vi "_LO_freq_Sweep_with_PM.vi"(9 "_LO_sweep":T3={"スケール"=200.0, "start (GHz)"=780.0, "stop (GHz)"=900.0, "step (GHz) "=0.1, "Wait(ms)"=10.0, "file_name"="", "パス"=path "", "measure"=0} {"measure" items=["SIS Current", "DMM34401A"]}, 10 "LO_misc":T1={"LO FRQ(GHz)"=900.0, "LO multi "=9.0, "LocK?"=FALSE, "LO REF multi"=4.0, "wait (ms)"=10.0, "SG Pow Min (dBm)"=10.0, "SG Pow Max (dBm)"=20.0, "SG Pow Step (dBm)"=0.2, "SGPow OPT? "=TRUE, "SG set frq"=25.0075, "SG set pow"=10.0}, 11 "Bias_LO_equip":T2={"Node address"=19, "CAN Interface"="CAN0", "Cartridge band"=10, "Slave Node in"={"Address"=19, "Serial Number"=[16, 71, 55, 76, 2, 8, 0, -15]}, "ObjHandle out"=159055936, "POL"=1, "sb"=1, "GPIB_SM (SIS S,V)"="24", "GPIB_DMM (SIS I)"="22", "GPIB_SM (MAG I) "="25", "GPIB_SG(LO)"="19", "GPIB_PW (PAMP) "="6", "GPIB_TMP1(8ch)"="12", "GPIB_TMP2(2ch)  "="13", "WCA_avg"=10, "Rsen"=10.0, "BiasModule"=0, "LOModule "=4, "WCA_LO_FREQ_SET"={"YTO Low freq. [GHz]"=14.42, "YTO High freq. [GHz]"=17.7, "Kvco"=1, "Lock Pol."=0, "SET LO FREQ"=72.5, "Multiplier"=6.0, "YTO (HEX)"=0, "YTO coarse( FREQ)"=25.0, "NULL PLL INTEGRATOR"=FALSE}} {"WCA_LO_FREQ_SET"."YTO coarse( FREQ)" min=25 max=150 step=0.0001 format="%.3f"; "WCA_LO_FREQ_SET"."Multiplier" min=3 max=6 step=3; "WCA_LO_FREQ_SET"."SET LO FREQ" min=25 max=150 step=0.0001 format="%.3f"; "WCA_LO_FREQ_SET"."Lock Pol." items=["Lower", "Upper"]; "WCA_LO_FREQ_SET"."Kvco" items=["7.5MHz/V", "15MHz/V"]; "WCA_LO_FREQ_SET"."YTO High freq. [GHz]" format="%.3f"; "WCA_LO_FREQ_SET"."YTO Low freq. [GHz]" format="%.3f"; "LOModule" items=["Manual Gunn+PAMP"=0, "B10Lab LO"=1, "WCA LO"=2, ""=3, "YIG発信器"=4, "none"=99]; "BiasModule" items=["B10Lab Bias"=0, "WCA BiasModule"=1, "none"=99]; "Slave Node in"."Serial Number" format="%.0x"; "Slave Node in"."Address" format="%.0x"; "Cartridge band" max=10 step=1; "Node address" format="%.0x"}) -> ()   [LabVIEW 2011]
uses:
  __sub_vi/WCA_NAOJ_sub_vi/WCA_Global.vi
panel:
  out "XYグラフ":cluster{dbl[], dbl[]}[](graph)
  in  "タブ制御器":enum32{"機器セッティング", "機器セッティング 2", "WCALOモニタ "}(tab)
  out "Link済み":bool
  out "error out":errorcluster={"status"=TRUE, "code"=-1074388991, "source"="NI-CAN Wait For State\n(ncWait.vi)"} caption="エラー出力"
  out "LO周波数":dbl=900.0
  out "出力":dbl=0.0096099853515625
  out "GET_PLL":T4={"PLL_ASSY_T"=37.887573, "PLL_REF_TOT_P"=-0.004119873, "PLL_IF_TOT_P"=0.010223389, "PLL_CORR_V"=0.08273038, "PLL_LOCK_V"=0.06496083, "PLL_5V_SUPPLY_V"=19.049072, "Temp_TF"=TRUE, "PLL Ref Pwr_TF"=FALSE, "IF Pwr_TF"=FALSE, "PLL Corr_TF"=TRUE, "PLL Lock V_TF"=FALSE, "PLL Nominal_TF"=FALSE}
  out "GET_AMC":T5={"AMC_A_DRAIN_V"=3.48938, "AMC_A_DRAIN_C"=64.42261, "AMC_A_GATE_V"=-0.4689026, "AMC_B_DRAIN_V"=4.34021, "AMC_B_DRAIN_C"=301.4679, "AMC_B_GATE_V"=-0.48934937, "AMC_E_DRAIN_V"=3.977356, "AMC_E_DRAIN_C"=342.6819, "AMC_E_GATE_V"=-0.24169922, "AMC_3V_SUPPLY_V"=-13.227844, "AMC_5V_MON"=5.204468, "AMC_MULT_D_V"=0.0}
  out "GET_PHOTOMIXER":T6={"PHOTMIX_ State"=enum."Disabled", "PHOTOMIX_BIAS_V"=-0.0012207031, "PHOTOMIX_BIAS_C"=-0.0032043457}
  out "GET_PA":T7={"PA_A_DRAIN_V"=4.0403748, "PA_A_DRAIN_C"=429.99268, "PA_A_GATE_V"=-0.00061035156, "PA_B_DRAIN_V"=0.0048828125, "PA_B_DRAIN_C"=2.5482178, "PA_B_GATE_V"=0.0015258789, "PA_3V_SUPPLY_V"=3.7130737, "PA_5V_MON"=5.3082275}
  # "LO freq. [GHz]"
  # "YTO LOW\n/High Freq."
  # "ZERO Intgrtr"
  # "Node Address"
  # "Serial Number"
  # "Vd [V]"
  # "Id [mA]"
  # "Vg [V]"
  # "AMC A"
  # "AMC B"
  # "AMC E"
  # "Vd [V]"
  # "Id [mA]"
  # "Vg [V]"
  # "PA -3V Supply"
  # "-3V"
  # "PA A"
  # "+5V"
  # "PA B"
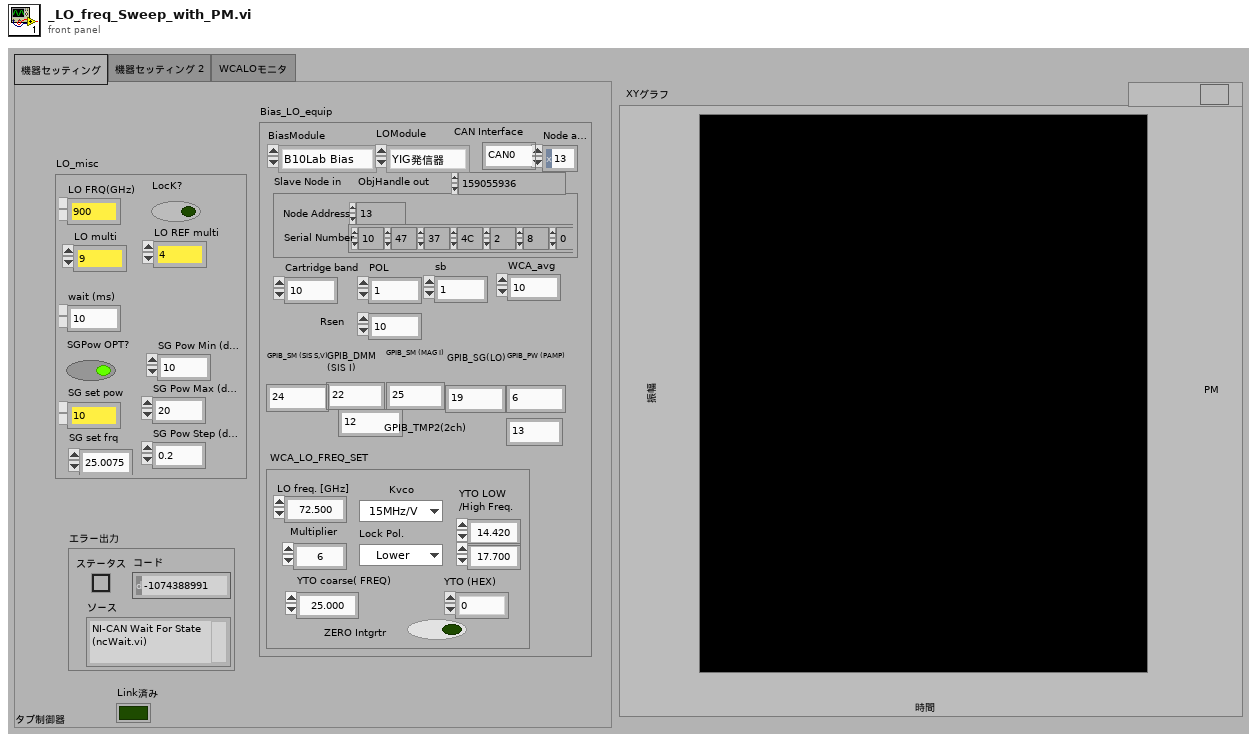
[diagram p1: front panel]
types:
  T1 = cluster{"LO FRQ(GHz)":dbl, "LO multi ":dbl, "LocK?":bool, "LO REF multi":dbl, "wait (ms)":dbl, "SG Pow Min (dBm)":dbl, "SG Pow Max (dBm)":dbl, "SG Pow Step (dBm)":dbl, "SGPow OPT? ":bool, "SG set frq":dbl, "SG set pow":dbl}
  T2 = cluster{"Node address":u16, "CAN Interface":string, "Cartridge band":u32, "Slave Node in":cluster{"Address":i16, "Serial Number":i8[]}, "ObjHandle out":u32, "POL":u32, "sb":u32, "GPIB_SM (SIS S,V)":string, "GPIB_DMM (SIS I)":string, "GPIB_SM (MAG I) ":string, "GPIB_SG(LO)":string, "GPIB_PW (PAMP) ":string, "GPIB_TMP1(8ch)":string, "GPIB_TMP2(2ch)  ":string, "WCA_avg":i32, "Rsen":dbl, "BiasModule":u16, "LOModule ":u16, "WCA_LO_FREQ_SET":cluster{"YTO Low freq. [GHz]":sgl, "YTO High freq. [GHz]":sgl, "Kvco":u16, "Lock Pol.":u16, "SET LO FREQ":sgl, "Multiplier":sgl, "YTO (HEX)":u16, "YTO coarse( FREQ)":sgl, "NULL PLL INTEGRATOR":bool}}
  T3 = cluster{"スケール":dbl, "start (GHz)":dbl, "stop (GHz)":dbl, "step (GHz) ":dbl, "Wait(ms)":dbl, "file_name":string, "パス":path, "measure":u16}
  T4 = cluster{"PLL_ASSY_T":sgl, "PLL_REF_TOT_P":sgl, "PLL_IF_TOT_P":sgl, "PLL_CORR_V":sgl, "PLL_LOCK_V":sgl, "PLL_5V_SUPPLY_V":sgl, "Temp_TF":bool, "PLL Ref Pwr_TF":bool, "IF Pwr_TF":bool, "PLL Corr_TF":bool, "PLL Lock V_TF":bool, "PLL Nominal_TF":bool}
  T5 = cluster{"AMC_A_DRAIN_V":sgl, "AMC_A_DRAIN_C":sgl, "AMC_A_GATE_V":sgl, "AMC_B_DRAIN_V":sgl, "AMC_B_DRAIN_C":sgl, "AMC_B_GATE_V":sgl, "AMC_E_DRAIN_V":sgl, "AMC_E_DRAIN_C":sgl, "AMC_E_GATE_V":sgl, "AMC_3V_SUPPLY_V":sgl, "AMC_5V_MON":sgl, "AMC_MULT_D_V":sgl}
  T6 = cluster{"PHOTMIX_ State":enum16{"Disabled", "Enabled"}, "PHOTOMIX_BIAS_V":sgl, "PHOTOMIX_BIAS_C":sgl}
  T7 = cluster{"PA_A_DRAIN_V":sgl, "PA_A_DRAIN_C":sgl, "PA_A_GATE_V":sgl, "PA_B_DRAIN_V":sgl, "PA_B_DRAIN_C":sgl, "PA_B_GATE_V":sgl, "PA_3V_SUPPLY_V":sgl, "PA_5V_MON":sgl}
  T8 = cluster{"Node address":u16, "CAN Interface":string, "Cartridge band":u32, "Slave Node in":cluster{"Address":i16, "Serial Number":i8[]}, "ObjHandle out":u32, "POL":u32, "sb":u32, "GPIB_SM (SIS S,V)":string, "GPIB_DMM (SIS I)":string, "GPIB_SM (MAG I) ":string, "GPIB_SG(LO)":string, "GPIB_PW (PAMP) ":string, "GPIB_TMP1(8ch)":string, "GPIB_TMP2(2ch)  ":string, "WCA_avg":i32, "Rsen":dbl, "BiasModule":u16, "LOModule ":u16, "WCA_LO_FREQ_SET":cluster{"YTO Low freq. [GHz]":sgl, "YTO High freq. [GHz]":sgl, "Kvco":u16, "Lock Pol.":u16, "SET LO FREQ":sgl, "Multiplier":sgl, "YTO (HEX)":u16, "YTO ( FREQ)":sgl, "NULL PLL INTEGRATOR":bool}}
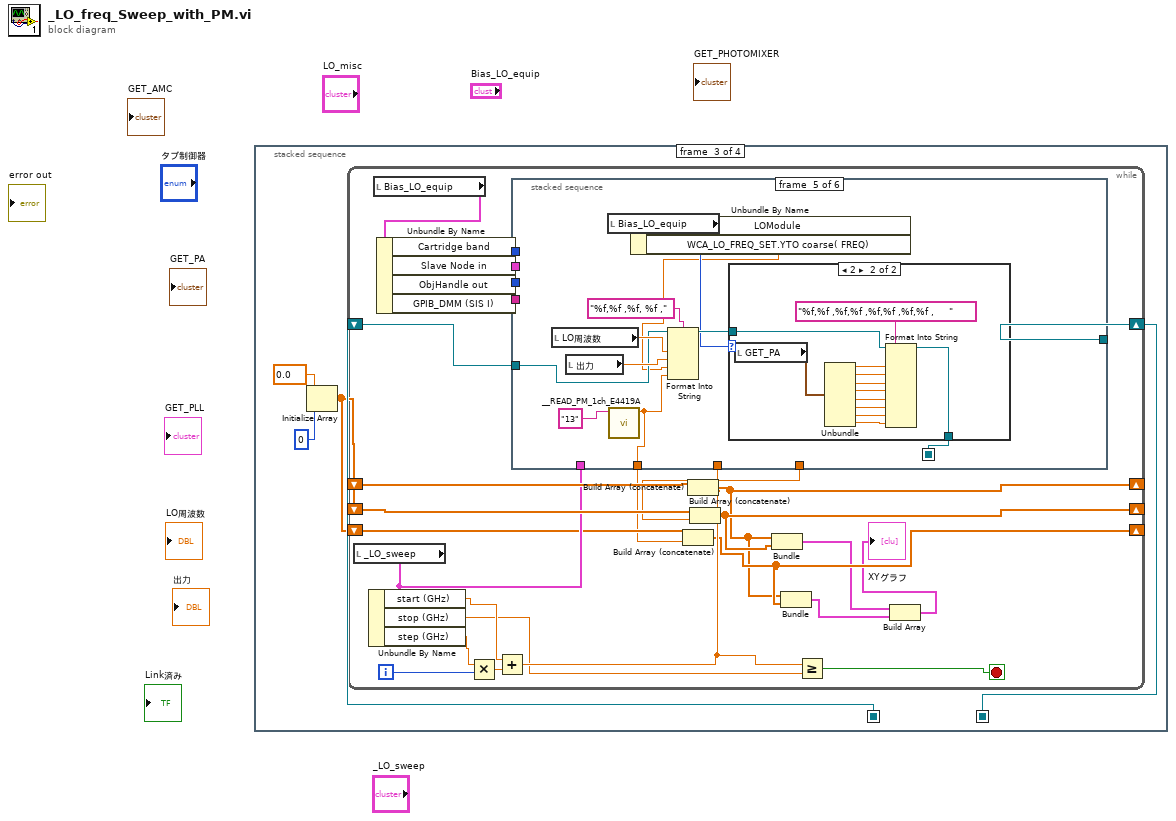
[diagram p0: block diagram]
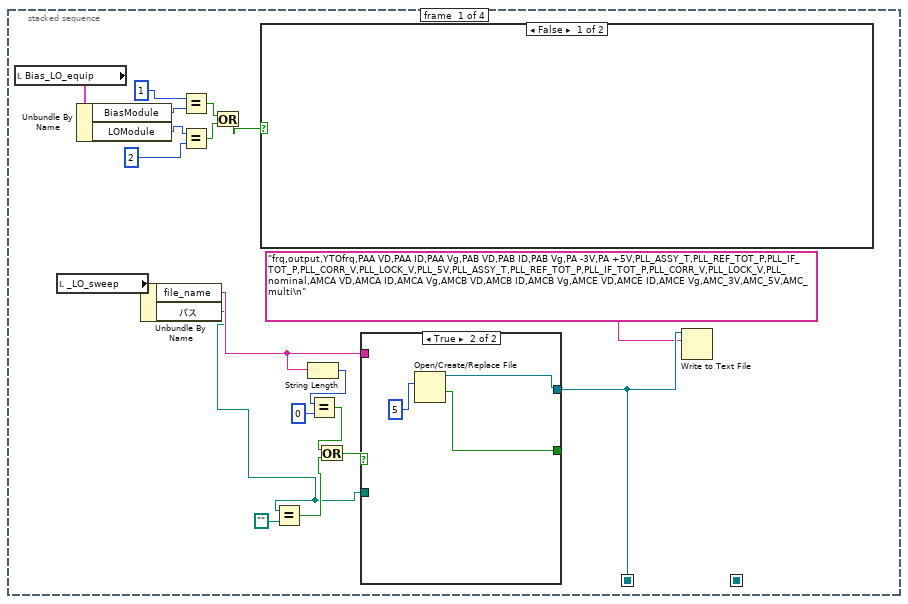
[diagram p2: hidden frame]
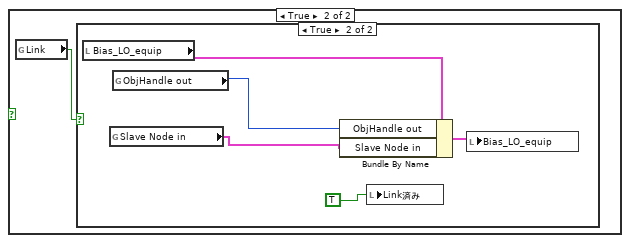
[diagram p3: hidden frame]
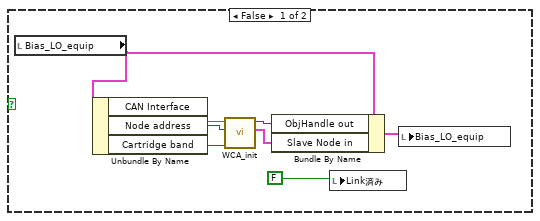
[diagram p4: hidden frame]
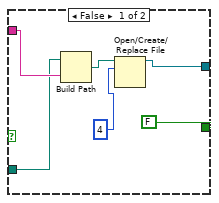
[diagram p5: hidden frame]
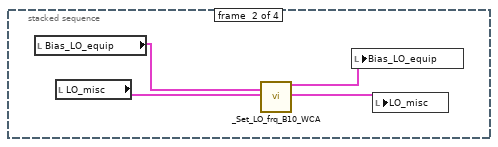
[diagram p6: hidden frame]
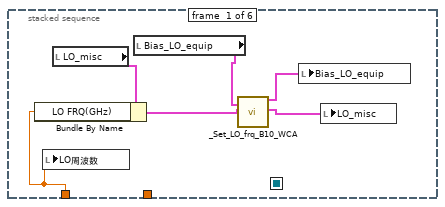
[diagram p7: hidden frame]
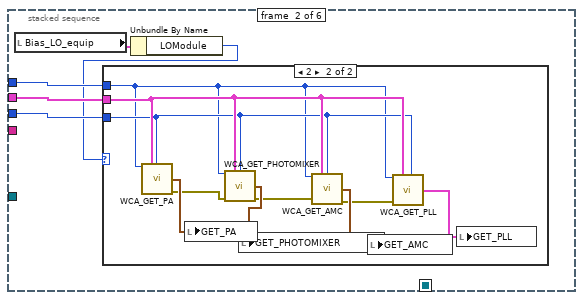
[diagram p8: hidden frame]
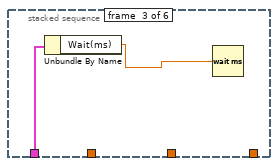
[diagram p10: hidden frame]
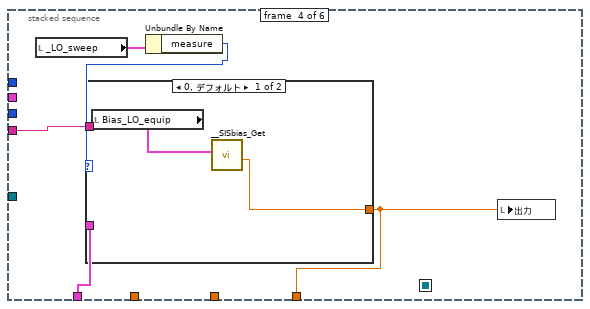
[diagram p11: hidden frame]
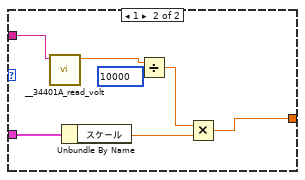
[diagram p12: hidden frame]
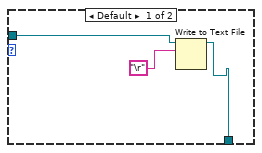
[diagram p13: hidden frame]
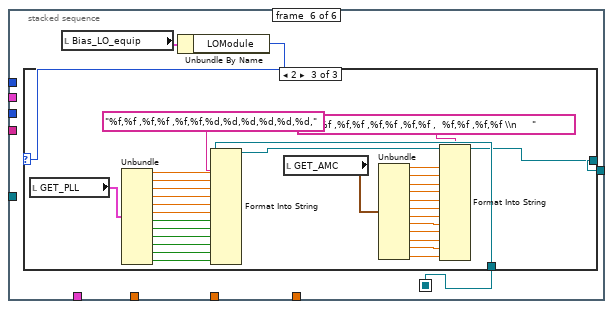
[diagram p14: hidden frame]
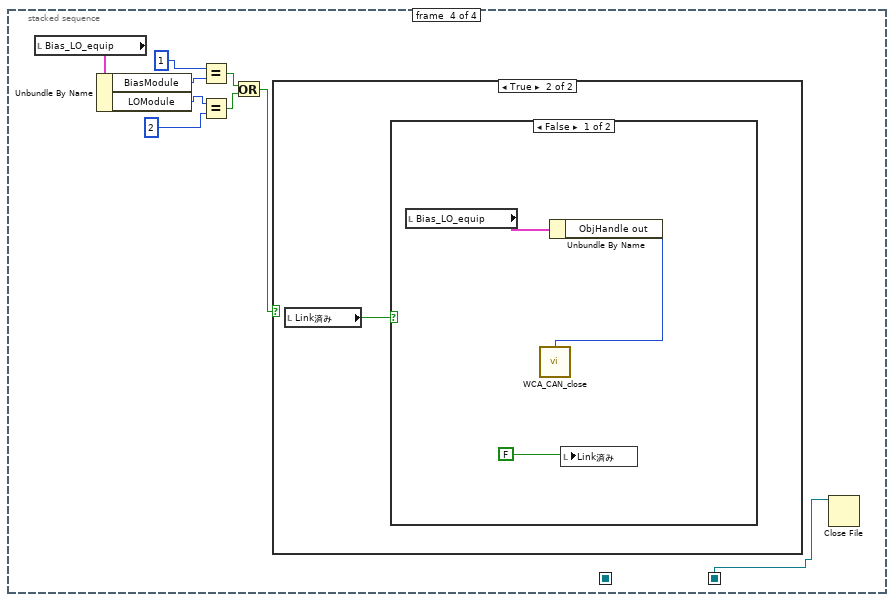
[diagram p17: hidden frame]
diagram:
  n1 = stacked-sequence {
    seq-local: [w13 _ _ _] -> [_ _ w49 _]
    seq-local: [_ _ w48 _] -> [_ _ _ w178]
    frame #0 {
      n2 = local read "Bias_LO_equip"() -> (w8:T2)
      n3 = local read "_LO_sweep"() -> (w11:T3)
      n4 = Unbundle By Name(w8) -> ("BiasModule"=w7:u16, "LOModule"=w5:u16)
      n5 = Unbundle By Name(w11) -> ("file_name"=w10:string, "パス"=w9:path)
      n6 = Equal?(x=1, y=w7) -> (x = y?=w3:bool)
      n7 = Equal?(x=w5, y=2) -> (x = y?=w2:bool)
      n8 = Or(x=w3, y=w2) -> (x .or. y?=w1:bool)
      n9 = case shown="FALSE" w1 {
        frame False {
        }
        frame True {
          n10 = global read "WCA_Global.vi" "Link"() -> (w20:bool)
          n11 = case shown="TRUE" w20 {
            frame False {
              n12 = local read "Bias_LO_equip"() -> (w22:T2)
              n13 = Unbundle By Name(w22) -> ("CAN Interface"=w26:string, "Node address"=w25:u16, "Cartridge band"=w24:u32)
              n14 = call "WCA_init.vi"("Cartridge band"=w24, "Node address"=w25, "CAN Interface"=w26) -> ("Slave Node in"=w27:cluster{"Address":i16, "Serial Number":i8[]}, "ObjHandle out"=w28:u32)  [unwired: 4 in, 3 out]
              n15 = Bundle By Name(cluster=w22, "ObjHandle out"=w28, "Slave Node in"=w27) -> (w23:T2)
              n16 = local write "Link済み"(FALSE) -> ()
              n17 = local write "Bias_LO_equip"(w23) -> ()
            }
            frame True {
              n18 = local read "Bias_LO_equip"() -> (w32:T2)
              n19 = global read "WCA_Global.vi" "Slave Node in"() -> (w30:cluster{"Address":i16, "Serial Number":i8[]})
              n20 = global read "WCA_Global.vi" "ObjHandle out"() -> (w31:u32)
              n21 = Bundle By Name(cluster=w32, "ObjHandle out"=w31, "Slave Node in"=w30) -> (w33:T2)
              n22 = local write "Link済み"(TRUE) -> ()
              n23 = local write "Bias_LO_equip"(w33) -> ()
            }
          }
        }
      }
      n24 = Equal?(x=w9, y=path "") -> (x = y?=w14:bool)
      n25 = String Length(string=w10) -> (length=w19:i32)
      n26 = Equal?(x=w19, y=0) -> (x = y?=w15:bool)
      n27 = Or(x=w15, y=w14) -> (x .or. y?=w16:bool)
      n28 = case shown="TRUE" w16 {
        tunnel: w10 -> [w39 _]
        tunnel: [w36 w40] -> w13
        tunnel: [FALSE w41] -> _
        tunnel: w9 -> [w37 _]
        frame False {
          n29 = Build Path(base path=w37, name or relative path=w39) -> (appended path=w35:path)
          n30 = Open/Create/Replace File(file path (use dialog)=w35, operation (0:open)=4) -> (refnum out=w36:refnum<file>)  [unwired: 4 in, 2 out]
        }
        frame True {
          n31 = Open/Create/Replace File(operation (0:open)=5) -> (refnum out=w40:refnum<file>, cancelled=w41:bool)  [unwired: 5 in, 1 out]
        }
      }
      n32 = Write to Text File(file (use dialog)=w13, text="frq,output,YTOfrq,PAA VD,PAA ID,PAA Vg,PAB VD,PAB ID,PAB Vg,PA -3V,PA +5V,PLL_ASSY_T,PLL_REF_TOT_P,PLL_IF_TOT_P,PLL_CORR_V,PLL_LOCK_V,PLL_5V,PLL_ASSY_T,PLL_REF_TOT_P,PLL_IF_TOT_P,PLL_CORR_V,PLL_LOCK_V,PLL_nominal,AMCA VD,AMCA ID,AMCA Vg,AMCB VD,AMCB ID,AMCB Vg,AMCE VD,AMCE ID,AMCE Vg,AMC_3V,AMC_5V,AMC_multi\n") -> ()  [unwired: 2 in, 3 out]
    }
    frame #1 {
      n33 = local read "Bias_LO_equip"() -> (w43:T2)
      n34 = local read "LO_misc"() -> (w46:T1)
      n35 = call "_Set_LO_frq_B10_WCA.vi"("Bias_LO_equip"=w43, "LO_misc"=w46) -> ("Bias_LO_equip 2"=w45:T8, "LO_misc 2"=w44:T1)  [unwired: 15 in, 1 out]
      n36 = local write "Bias_LO_equip"(w45) -> ()
      n37 = local write "LO_misc"(w44) -> ()
    }
    frame #2 {
      n38 = Initialize Array(0.0, 0) -> (w47:dbl[])
      n39 = while {
        shift-right: [w52] -> _
        shift-left: w47 -> [w70]
        shift-right: [w68] -> _
        shift-left: w47 -> [w69]
        shift-right: [w64] -> w48
        shift-left: w49 -> [w65]
        shift-right: [w56] -> _
        shift-left: w47 -> [w58]
        i -> [w77]
        stop <- w75 stop-if-true
        n40 = local read "_LO_sweep"() -> (w60:T3)
        n41 = Unbundle By Name(w60) -> ("start (GHz)"=w63:dbl, "stop (GHz)"=w61:dbl, "step (GHz)"=w62:dbl)
        n42 = local read "Bias_LO_equip"() -> (w59:T2)
        n43 = Unbundle By Name(w59) -> ("Cartridge band"=w72:u32, "Slave Node in"=w73:cluster{"Address":i16, "Serial Number":i8[]}, "ObjHandle out"=w74:u32, "GPIB_DMM (SIS I)"=w71:string)
        n44 = Multiply(x=w62, y=w77) -> (x*y=w76:dbl)
        n45 = Add(x=w63, y=w76) -> (x+y=w67:dbl)
        n46 = stacked-sequence {
          seq-local: [_ _ _ _ w120 _] -> [_ _ _ _ _ w144]
          tunnel: w67 -> [w83 _ _ _ _ _]
          tunnel: w74 -> [_ w87 _ _ _ _]
          tunnel: w73 -> [_ w88 _ _ _ _]
          tunnel: w72 -> [_ w86 _ _ _ _]
          tunnel: w71 -> [_ _ _ w101 _ _]
          tunnel: [_ _ _ w105 _ _] -> w66
          tunnel: w65 -> [_ _ _ _ w122 _]
          tunnel: [_ _ _ _ _ w143] -> w64
          tunnel: w60 -> [_ _ w100 w104 _ _]
          tunnel: [_ _ _ _ w115 _] -> w57
          frame #0 {
            n47 = local write "LO周波数"(w83) -> ()
            n48 = local read "LO_misc"() -> (w82:T1)
            n49 = Bundle By Name(cluster=w82, "LO FRQ(GHz)"=w83) -> (w81:T1)
            n50 = local read "Bias_LO_equip"() -> (w78:T2)
            n51 = call "_Set_LO_frq_B10_WCA.vi"("Bias_LO_equip"=w78, "LO_misc"=w81) -> ("Bias_LO_equip 2"=w80:T8, "LO_misc 2"=w79:T1)  [unwired: 15 in, 1 out]
            n52 = local write "Bias_LO_equip"(w80) -> ()
            n53 = local write "LO_misc"(w79) -> ()
          }
          frame #1 {
            n54 = local read "Bias_LO_equip"() -> (w85:T2)
            n55 = Unbundle By Name(w85) -> ("LOModule"=w84:u16)
            n56 = case shown="2" w84 {
              tunnel: w88 -> [_ w94]
              tunnel: w87 -> [_ w93]
              tunnel: w86 -> [_ w92]
              frame 0, Default {
              }
              frame 2 {
                n57 = call "WCA_GET_PA.vi"("Cartridge Band"=w92, "Slave Node in"=w94, "ObjHandle in"=w93) -> ("GET_PA"=w95:T7, "error out"=w91:errorcluster)  [unwired: 10 in, 1 out]
                n58 = local write "GET_PA"(w95) -> ()
                n59 = call "WCA_GET_PHOTOMIXER.vi"("Cartridge Band"=w92, "Slave Node in"=w94, "ObjHandle in"=w93, "error in (no error)"=w91) -> ("GET_PHOTOMIXER"=w97:T6, "error out"=w90:errorcluster)  [unwired: 9 in, 1 out]
                n60 = local write "GET_PHOTOMIXER"(w97) -> ()
                n61 = call "WCA_GET_AMC.vi"("Cartridge Band"=w92, "Slave Node in"=w94, "ObjHandle in"=w93, "error in (no error)"=w90) -> ("GET_AMC"=w98:T5, "error out"=w89:errorcluster)  [unwired: 9 in, 1 out]
                n62 = local write "GET_AMC"(w98) -> ()
                n63 = call "WCA_GET_PLL.vi"("Cartridge Band"=w92, "Slave Node in"=w94, "ObjHandle in"=w93, "error in (no error)"=w89) -> ("GET_PLL"=w96:T4)  [unwired: 9 in, 2 out]
                n64 = local write "GET_PLL"(w96) -> ()
              }
            }
          }
          frame #2 {
            n65 = Unbundle By Name(w100) -> ("Wait(ms)"=w99:dbl)
            n66 = Wait (ms)(milliseconds to wait=w99) -> ()  [unwired: 1 out]
          }
          frame #3 {
            n67 = local read "_LO_sweep"() -> (w103:T3)
            n68 = Unbundle By Name(w103) -> ("measure"=w102:u16)
            n69 = case shown="0, デフォルト" w102 {
              tunnel: [w106 w111] -> w105
              tunnel: w104 -> [_ w110]
              tunnel: w101 -> [_ w108]
              frame 0, Default {
                n70 = local read "Bias_LO_equip"() -> (w107:T2)
                n71 = call "__SISbias_Get.vi"("Bias_LO_equip"=w107) -> ("Get_I(uA)"=w106:dbl)  [unwired: 8 in, 2 out]
              }
              frame 1 {
                n72 = call "__34401A_read_volt.vi"("GPIB"=w108) -> ("Read_volt(mV)"=w113:dbl)  [unwired: 6 in]
                n73 = Unbundle By Name(w110) -> ("スケール"=w109:dbl)
                n74 = Divide(x=w113, y=10000) -> (x/y=w114:dbl)
                n75 = Multiply(x=w114, y=w109) -> (x*y=w111:dbl)
              }
            }
            n76 = local write "出力"(w105) -> ()
          }
          frame #4 {
            n77 = local read "LO周波数"() -> (w124:dbl)
            n78 = local read "出力"() -> (w123:dbl)
            n79 = local read "Bias_LO_equip"() -> (w119:T2)
            n80 = call "__READ_PM_1ch_E4419A.VI"("GPIB"="13") -> ("chA"=w115:dbl)  [unwired: 6 in]
            n81 = Unbundle By Name(w119) -> ("LOModule"=w118:u16, "WCA_LO_FREQ_SET.YTO coarse( FREQ)"=w117:sgl)
            n82 = Format Into String(format string="%f,%f ,%f, %f ,", initial string=w122, w124, w123, w117, w115) -> (resulting string=w121:refnum<file>)  [unwired: 1 in, 1 out]
            n83 = case shown="2" w118 {
              tunnel: w121 -> [w127 w130]
              tunnel: [w128 w129] -> w120
              frame Default {
                n84 = Write to Text File(file (use dialog)=w127, text="\r") -> (refnum out=w128:refnum<file>)  [unwired: 2 in, 2 out]
              }
              frame 2 {
                n85 = local read "GET_PA"() -> (w140:T7)
                n86 = Unbundle(w140) -> ("PA_A_DRAIN_V"=w138:sgl, "PA_A_DRAIN_C"=w137:sgl, "PA_A_GATE_V"=w136:sgl, "PA_B_DRAIN_V"=w135:sgl, "PA_B_DRAIN_C"=w134:sgl, "PA_B_GATE_V"=w133:sgl, "PA_3V_SUPPLY_V"=w132:sgl, "PA_5V_MON"=w131:sgl)
                n87 = Format Into String(format string="%f,%f ,%f,%f ,%f,%f ,%f,%f ,     ", initial string=w130, w138, w137, w136, w135, w134, w133, w132, w131) -> (resulting string=w129:refnum<file>)  [unwired: 1 in, 1 out]
              }
            }
          }
          frame #5 {
            n88 = local read "Bias_LO_equip"() -> (w142:T2)
            n89 = Unbundle By Name(w142) -> ("LOModule"=w141:u16)
            n90 = case shown="2" w141 {
              tunnel: w144 -> [w145 w146 w154]
              tunnel: [w145 w146 w152] -> w143
              frame 0, Default {
              }
              frame 1 {
              }
              frame 2 {
                n91 = local read "GET_PLL"() -> (w177:T4)
                n92 = Unbundle(w177) -> ("PLL_ASSY_T"=w175:sgl, "PLL_REF_TOT_P"=w174:sgl, "PLL_IF_TOT_P"=w173:sgl, "PLL_CORR_V"=w172:sgl, "PLL_LOCK_V"=w171:sgl, "PLL_5V_SUPPLY_V"=w170:sgl, "Temp_TF"=w169:bool, "PLL Ref Pwr_TF"=w168:bool, "IF Pwr_TF"=w167:bool, "PLL Corr_TF"=w166:bool, "PLL Lock V_TF"=w165:bool, "PLL Nominal_TF"=w164:bool)
                n93 = Format Into String(format string="%f,%f ,%f,%f ,%f,%f,%d,%d,%d,%d,%d,%d,", initial string=w154, w175, w174, w173, w172, w171, w170, w169, w168, w167, w166, w165, w164) -> (resulting string=w153:refnum<file>)  [unwired: 1 in, 1 out]
                n94 = local read "GET_AMC"() -> (w155:T5)
                n95 = Unbundle(w155) -> ("AMC_A_DRAIN_V"=w156:sgl, "AMC_A_DRAIN_C"=w157:sgl, "AMC_A_GATE_V"=w158:sgl, "AMC_B_DRAIN_V"=w159:sgl, "AMC_B_DRAIN_C"=w160:sgl, "AMC_B_GATE_V"=w161:sgl, "AMC_E_DRAIN_V"=w162:sgl, "AMC_E_DRAIN_C"=w163:sgl, "AMC_E_GATE_V"=w151:sgl, "AMC_3V_SUPPLY_V"=w150:sgl, "AMC_5V_MON"=w149:sgl, "AMC_MULT_D_V"=w148:sgl)
                n96 = Format Into String(format string="%f,%f ,%f,%f ,%f,%f ,%f,%f ,  %f,%f ,%f,%f \\n     ", initial string=w153, w156, w157, w158, w159, w160, w161, w162, w163, w151, w150, w149, w148) -> (resulting string=w152:refnum<file>)  [unwired: 1 in, 1 out]
              }
            }
          }
        }
        n97 = Build Array (concatenate)(w58, w57) -> (w56:dbl[])
        n98 = Build Array (concatenate)(w70, w67) -> (w52:dbl[])
        n99 = Build Array (concatenate)(w69, w66) -> (w68:dbl[])
        n100 = Bundle(w52, w68) -> (w55:cluster{dbl[], dbl[]})  [unwired: 1 in]
        n101 = Bundle(w52, w56) -> (w54:cluster{dbl[], dbl[]})  [unwired: 1 in]
        n102 = Greater Or Equal?(x=w67, y=w61) -> (x >= y?=w75:bool)
        n103 = Build Array(w55, w54) -> (→"XYグラフ":cluster{dbl[], dbl[]}[])
      }
    }
    frame #3 {
      n104 = local read "Bias_LO_equip"() -> (w186:T2)
      n105 = Unbundle By Name(w186) -> ("BiasModule"=w185:u16, "LOModule"=w183:u16)
      n106 = Equal?(x=1, y=w185) -> (x = y?=w181:bool)
      n107 = Equal?(x=w183, y=2) -> (x = y?=w180:bool)
      n108 = Or(x=w181, y=w180) -> (x .or. y?=w179:bool)
      n109 = case shown="TRUE" w179 {
        frame False {
        }
        frame True {
          n110 = local read "Link済み"() -> (w187:bool)
          n111 = case shown="FALSE" w187 {
            frame False {
              n112 = local read "Bias_LO_equip"() -> (w189:T2)
              n113 = Unbundle By Name(w189) -> ("ObjHandle out"=w188:u32)
              n114 = call "WCA_CAN_close.vi"("ObjHandle in"=w188) -> ()  [unwired: 14 in, 1 out]
              n115 = local write "Link済み"(FALSE) -> ()
            }
            frame True {
            }
          }
        }
      }
      n116 = Close File(refnum=w178) -> ()  [unwired: 1 in, 2 out]
    }
  }
